vi "(SubVI) Record Options for DRC.vi"(4 "Enum":T1(ring)) -> (1 "Record options":i32)   [LabVIEW 2014]
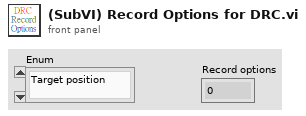
[diagram p1: front panel]
types:
  T1 = enum16{"Target position", "Current position", "position error"}
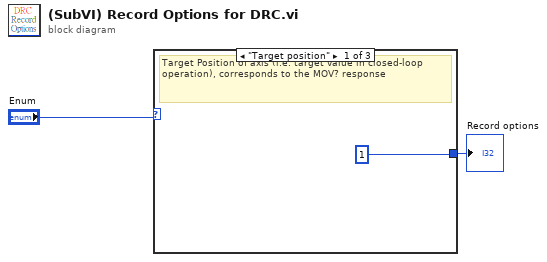
[diagram p0: block diagram]
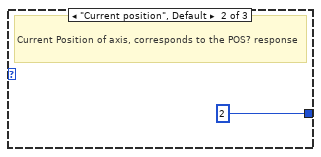
[diagram p2: hidden frame]
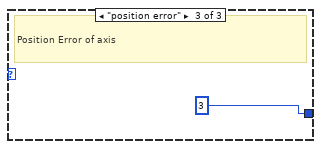
[diagram p3: hidden frame]
diagram:
  n1 = case shown="\"Target position\"" "Enum" {
    tunnel: [1 2 3] -> w1
    frame "Target position" {
      # "Target Position of axis (i.e. target value in closed-loop operation), corresponds to the MOV? response"
    }
    frame "Current position", Default {
      # "Current Position of axis, corresponds to the POS? response"
    }
    frame "position error" {
      # "Position Error of axis"
    }
  }
  "Record options" <- w1
